vi "Get Path Regex.vi"(8 "error in (no error)":errorcluster, 11 "TimerActionController in":refnum<class "TimerActionController.lvclass">) -> (0 "error out":errorcluster, 2 "Path Regex":string, 3 "TimerActionController out":refnum<class "TimerActionController.lvclass">)   [LabVIEW 2020, in "Timer Demo.lvlib" / "TimerActionController.lvclass"]
uses:
  TimerActionController.lvclass
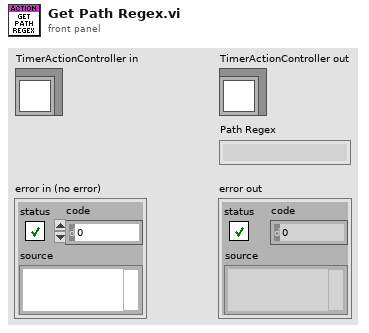
[diagram p1: front panel]
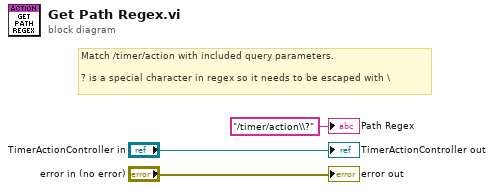
[diagram p0: block diagram]
diagram:
  # "Match /timer/action with included query parameters.\n\n? is a special character in regex so it needs to be escaped with \\"
  "error out" <- "error in (no error)"
  "TimerActionController out" <- "TimerActionController in"
  "Path Regex" <- "/timer/action\\?" ("Path Regex")
